vi "APS set gantry axis.vi"(7 "Slave_Axis_ID":i32, 8 "error in (no error)":errorcluster caption="错误输入（无错误）", 9 "Master_Axis_ID":i32, 10 "GroupNum":i32, 11 "Board_ID":i32) -> (0 "error out":errorcluster caption="错误输出", 3 "function return":i32)   [LabVIEW 2011, in "APS168.lvlib"]
doc: "I32 FNTYPE APS_set_gantry_axis( I32 Board_ID, I32 GroupNum, I32 Master_Axis_ID, I32 Slave_Axis_ID );"
uses:
  APS168.lvlib
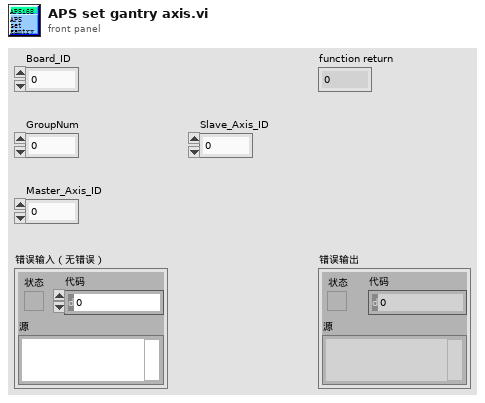
[diagram p1: front panel]
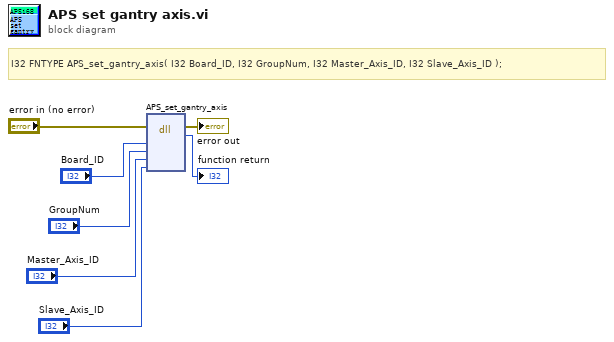
[diagram p0: block diagram]
diagram:
  # "I32 FNTYPE APS_set_gantry_axis( I32 Board_ID, I32 GroupNum, I32 Master_Axis_ID, I32 Slave_Axis_ID );"
  n1 = dll-call lib="PTH1Labs E软件ADLINK 204CAPS_1_7_1_LIB line 连续运动204APS168.*" fn="APS_set_gantry_axis"(error in="error in (no error)", "Board_ID"="Board_ID", "GroupNum"="GroupNum", "Master_Axis_ID"="Master_Axis_ID", "Slave_Axis_ID"="Slave_Axis_ID") -> (error out=→"error out":errorcluster, →"function return":i32)  [unwired: 6 in, 1 out]
